vi "Test Tokenizer Error Generation.vi"(8 "error in (no error)":errorcluster) -> (0 "error out":errorcluster)   [LabVIEW 2019]
uses:
  PathTokenizer/PathTokenizer.lvclass
  <vilib>/addons/_JKI Toolkits/Caraya/classes/Assert/Assert Error.vi
  <vilib>/addons/_JKI Toolkits/Caraya/classes/Test/Test.lvclass
  <vilib>/addons/_JKI Toolkits/Caraya/classes/Assert/Assert.lvclass
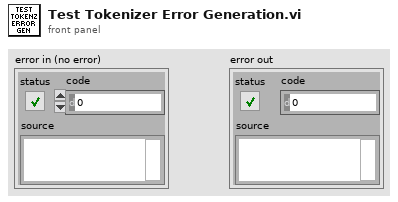
[diagram p1: front panel]
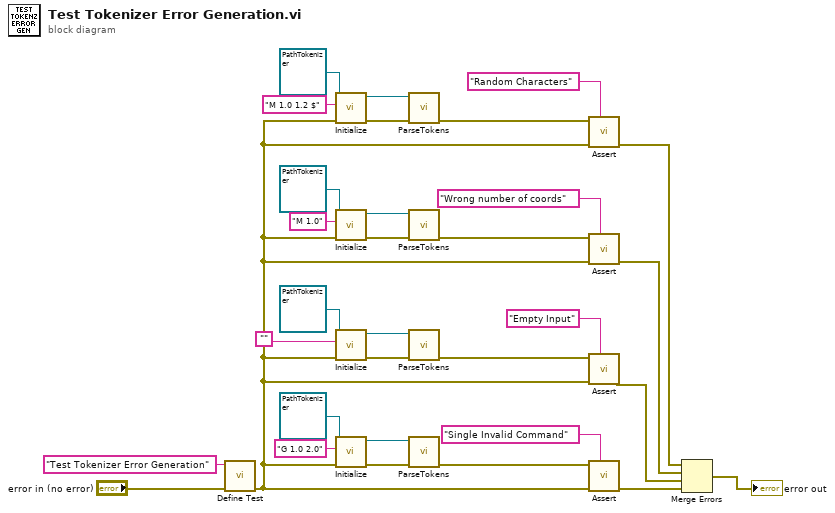
[diagram p0: block diagram]
diagram:
  n1 = call <vilib>:"Define Test.vi"("error in (no error)"="error in (no error)", "Label (VI Title)"="Test Tokenizer Error Generation") -> ("error out"=w2:errorcluster)  [unwired: 8 in, 1 out]
  n2 = call "Initialize.vi"("error in (no error)"=w2, "Path Command Text"="M 1.0 1.2 $", "PathTokenizer in"=refnum<class "PathTokenizer.lvclass"> refnum) -> ("error out"=w5:errorcluster, "PathTokenizer out"=w6:refnum<class "PathTokenizer.lvclass">)  [unwired: 7 in]
  n3 = call "Initialize.vi"("error in (no error)"=w2, "Path Command Text"="M 1.0", "PathTokenizer in"=refnum<class "PathTokenizer.lvclass"> refnum) -> ("error out"=w13:errorcluster, "PathTokenizer out"=w12:refnum<class "PathTokenizer.lvclass">)  [unwired: 7 in]
  n4 = call "Initialize.vi"("error in (no error)"=w2, "Path Command Text"="", "PathTokenizer in"=refnum<class "PathTokenizer.lvclass"> refnum) -> ("error out"=w19:errorcluster, "PathTokenizer out"=w21:refnum<class "PathTokenizer.lvclass">)  [unwired: 7 in]
  n5 = call "Initialize.vi"("error in (no error)"=w2, "Path Command Text"="G 1.0 2.0", "PathTokenizer in"=refnum<class "PathTokenizer.lvclass"> refnum) -> ("error out"=w27:errorcluster, "PathTokenizer out"=w28:refnum<class "PathTokenizer.lvclass">)  [unwired: 7 in]
  n6 = call "ParseTokens.vi"("error in (no error)"=w5, "PathTokenizer in"=w6) -> ("error out"=w3:errorcluster)  [unwired: 8 in, 1 out]
  n7 = call "ParseTokens.vi"("error in (no error)"=w13, "PathTokenizer in"=w12) -> ("error out"=w15:errorcluster)  [unwired: 8 in, 1 out]
  n8 = call "ParseTokens.vi"("error in (no error)"=w19, "PathTokenizer in"=w21) -> ("error out"=w17:errorcluster)  [unwired: 8 in, 1 out]
  n9 = call "ParseTokens.vi"("error in (no error)"=w27, "PathTokenizer in"=w28) -> ("error out"=w26:errorcluster)  [unwired: 8 in, 1 out]
  n10 = call-poly <vilib>:"Assert.vi"("Label"="Random Characters", "error in (no error)"=w2, "Error?"=w3) -> ("error out"=w1:errorcluster)  [unwired: 7 in, 1 out]
  n11 = call-poly <vilib>:"Assert.vi"("Label"="Wrong number of coords", "error in (no error)"=w2, "Error?"=w15) -> ("error out"=w9:errorcluster)  [unwired: 7 in, 1 out]
  n12 = call-poly <vilib>:"Assert.vi"("Label"="Empty Input", "error in (no error)"=w2, "Error?"=w17) -> ("error out"=w16:errorcluster)  [unwired: 7 in, 1 out]
  n13 = call-poly <vilib>:"Assert.vi"("Label"="Single Invalid Command", "error in (no error)"=w2, "Error?"=w26) -> ("error out"=w29:errorcluster)  [unwired: 7 in, 1 out]
  n14 = Merge Errors(w1, w9, w16, w29) -> (→"error out":errorcluster)
